vi "VMS_3_Responder.vi"() -> ()   [LabVIEW 2018]
uses:
  <vilib>/rvi/Emulation/niFpgaGetClockAttributes.vi
  <vilib>/rvi/Emulation/niFpgaSctlEmulationGetInTimedLoop.vi
  <vilib>/rvi/Emulation/niFpgaEmulationReportErrorSimple.vi
  <vilib>/rvi/eio/common/nirviEmuTemplateMethod_errors.vi
  <vilib>/rvi/DataTransferAndStorage/Container/Common/niFpgaContainerGetUniqueNameForEmu.vi
  <vilib>/rvi/DataTransferAndStorage/Container/Common/niFpgaContainerSetEmuInfo.vi
  <vilib>/rvi/eio/common/nirviEmuReportErrorAndStop.vi
  <vilib>/rvi/DataTransferAndStorage/Container/Common/niFpgaContainerExecOnDevCompGetState.vi
  <vilib>/rvi/Emulation/niFpgaEmulationIsFPGAContextNoSignature.vi
  <vilib>/rvi/Memory/Memory_Emulation/niFpgaMemoryEmulationCacheClearOnFirstRun.vi
  <vilib>/rvi/Memory/Memory_Emulation/nirvimemoryEmulationManagerCache_MakeExclusive.vi
  <vilib>/rvi/Memory/Memory_Emulation/niFpgaMemoryEmulationValidateCache.vi
  <vilib>/rvi/Memory/Memory_Emulation/nirvimemoryEmulationManagerCache_InsertValue.vi
  <vilib>/Utility/error.llb/Clear Errors.vi
  <vilib>/rvi/Memory/Memory_Emulation/nirvimemoryEmulationManagerCache_ReleaseExclusive.vi
  <vilib>/rvi/Memory/Memory_Emulation/nirvimemoryEmulationManagerCache_GetValue.vi
  <vilib>/rvi/Memory/Memory_Emulation/nirvimemoryEmulationManagerCache_SetValue.vi
  <vilib>/rvi/Emulation/niFpgaProcessEmulError.vi
  <vilib>/rvi/Emulation/niFpgaCriticalErrorInLSC.vi
  <vilib>/rvi/occurrence/nirviWaitOnOccurrenceBase.vi
  <vilib>/eio/EIONode/EIONode.xnode
  <vilib>/rvi/LocalResourceManager/LocalResourceManager.xnode
  <vilib>/rvi/DataTransferAndStorage/Container/XNode/niFpgaContainer.xnode
  <vilib>/rvi/DataTransferAndStorage/Register/Emulation/niFpgaRegisterEmulationRefIn.vi
  <vilib>/eio/EIOMethodNode/EIOMethodNode.xnode
panel:
  out "Stopped":bool
  in  "Timeout":i32=-1
  out "Timeouted":bool
  out "Ticks":u64
  out "Ready":bool
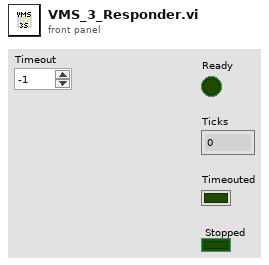
[diagram p1: front panel]
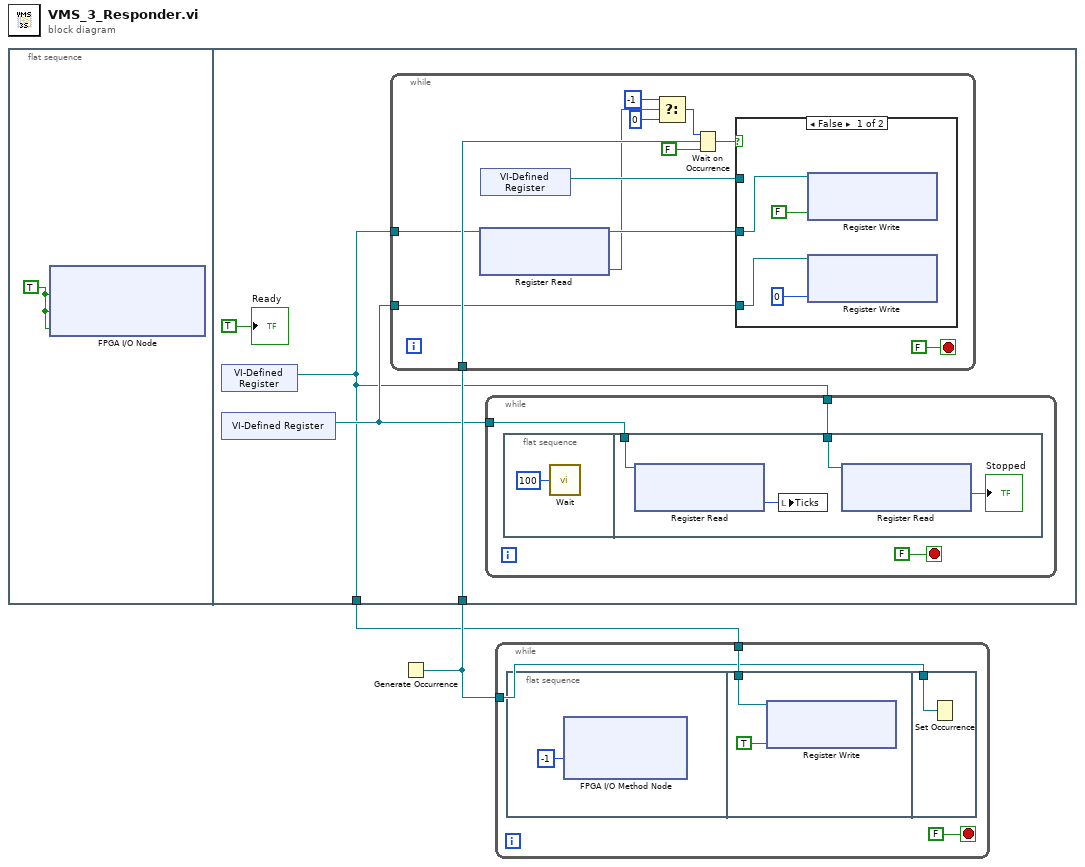
[diagram p0: block diagram]
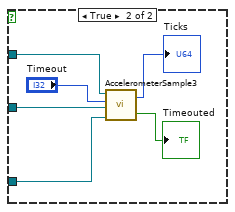
[diagram p2: hidden frame]
diagram:
  n1 = flat-sequence {
    tunnel: w2 -> [w6]
    tunnel: [w4] -> w1
    frame #0 {
      w3 = TRUE ("Accelerometer5/Start")
      n2 = xnode "FPGA I/O Node"("Accelerometer1/Start"=w3, "Accelerometer2/Start"=w3, "Accelerometer3/Start"=w3) -> ()  [unwired: 3 in, 3 out]
    }
    frame #1 {
      n3 = xnode "VI-Defined Register"() -> ("Register Out"=w4:refnum<k21>)
      n4 = xnode "VI-Defined Register"() -> ("Register Out"=w5:refnum<k21>)
      n5 = while {
        tunnel: w6 -> [w25]
        tunnel: w4 -> [w23]
        tunnel: w5 -> [w22]
        stop <- FALSE stop-if-true
        n6 = xnode ("Register Read")("Register In"=w23) -> ("Data"=w16:bool, "Register Out"=w21:refnum<k21>)
        n7 = xnode "VI-Defined Register"() -> ("Register Out"=w24:refnum<k21>)
        n8 = Select(t=-1, s=w16, f=0) -> (s? t:f=w19:i32)
        n9 = Wait on Occurrence(1:FALSE ("ignore previous (T)"), 2:w25, 3:w19) -> (0:w26:bool)
        n10 = case shown="False" w26 {
          tunnel: w22 -> [w31 w37]
          tunnel: w24 -> [_ w35]
          tunnel: w21 -> [w29 w36]
          frame False {
            n11 = xnode ("Register Write")("Data"=FALSE, "Register In"=w29) -> ()  [unwired: 1 out]
            n12 = xnode ("Register Write")("Data"=u64 0, "Register In"=w31) -> ()  [unwired: 1 out]
          }
          frame True {
            n13 = call "AccelerometerSample3.vi"("Ticks register"=w37, "Stop"=w36, "Timeout"="Timeout", "Output"=w35) -> ("Timeouted"=→"Timeouted":bool, "Ticks"=→"Ticks":u64)
          }
        }
      }
      n14 = while {
        tunnel: w5 -> [w9]
        tunnel: w4 -> [w8]
        stop <- FALSE stop-if-true
        n15 = flat-sequence {
          tunnel: w9 -> [w15]
          tunnel: w8 -> [w13]
          frame #0 {
            n16 = call "Wait"("Count(mSec)"=u32 100) -> ()  [unwired: 1 out]
          }
          frame #1 {
            n17 = xnode ("Register Read")("Register In"=w15) -> ("Data"=w14:u64)  [unwired: 1 out]
            n18 = local write "Ticks"(w14) -> ()
            n19 = xnode ("Register Read")("Register In"=w13) -> ("Data"=→"Stopped":bool)  [unwired: 1 out]
          }
        }
      }
      "Ready" <- TRUE ("Ready")
    }
  }
  n20 = Generate Occurrence() -> (w2:refnum<k4>)
  n21 = while {
    tunnel: w2 -> [w38]
    tunnel: w1 -> [w39]
    stop <- FALSE stop-if-true
    n22 = flat-sequence {
      tunnel: w39 -> [w43]
      tunnel: w38 -> [w44]
      frame #0 {
        n23 = xnode "FPGA I/O Method Node"("Timeout"=-1) -> ()  [unwired: 1 in, 2 out]
      }
      frame #1 {
        n24 = xnode ("Register Write")("Data"=TRUE, "Register In"=w43) -> ()  [unwired: 1 out]
      }
      frame #2 {
        n25 = Set Occurrence(w44) -> ()
      }
    }
  }
